vi "五参数水样测试.vi"(11 "启动参数":T1={"测量模式"="", "数据类型"="N"}) -> ()   [LabVIEW 2016, in "斯坦道原位多参数.lvlib"]
panel:
  in  "水温数据时间":timestamp
  out "Elapsed Time (s)":dbl caption="已用时间(s)"
  out "状态":string
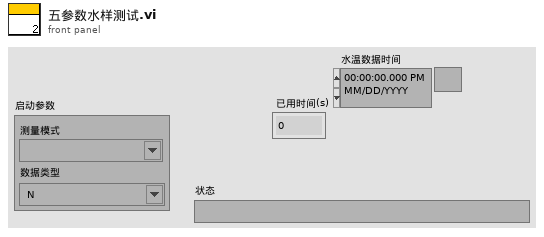
[diagram p1: front panel]
types:
  T1 = typedef "斯坦道原位多参数.lvlib/水样测试启动自定义输入参数.ctl" = cluster{"测量模式":string, "数据类型":string}
  T2 = cluster{"时间标识":timestamp, "设备":string, "日志信息":string, "流程参数":string}
  T3 = cluster{"水温":bool, "pH":bool, "DO":bool, "DOper":bool, "电导率":bool, "ORP":bool, "浊度":bool, "叶绿素a":bool, "藻密度":bool, "蓝绿藻":bool}
  T4 = typedef "原位多参数全参数字段定义.ctl" = cluster{"时间":timestamp, "水温":dbl, "pH":dbl, "DO":dbl, "DO%":dbl, "电导率":dbl, "ORP":dbl, "浊度":dbl, "叶绿素a":dbl, "藻密度":dbl, "蓝绿藻":dbl}
  T5 = cluster{"因子编码":string, "单位":string, "标样参考值":sgl, "水样数据时间":timestamp, "水样实测值":sgl, "水样数据标识":string, "K":sgl, "B":sgl, "T":sgl, "H":sgl, "水深":sgl, "探头温度":sgl, "信号值":sgl}
  T6 = cluster{"水温":dbl, "pH":dbl, "DO":dbl, "Cond":dbl, "Turb":dbl, "叶绿素":dbl, "藻密度":dbl, "蓝绿藻":dbl, "ORP":dbl, "NH3N":dbl}
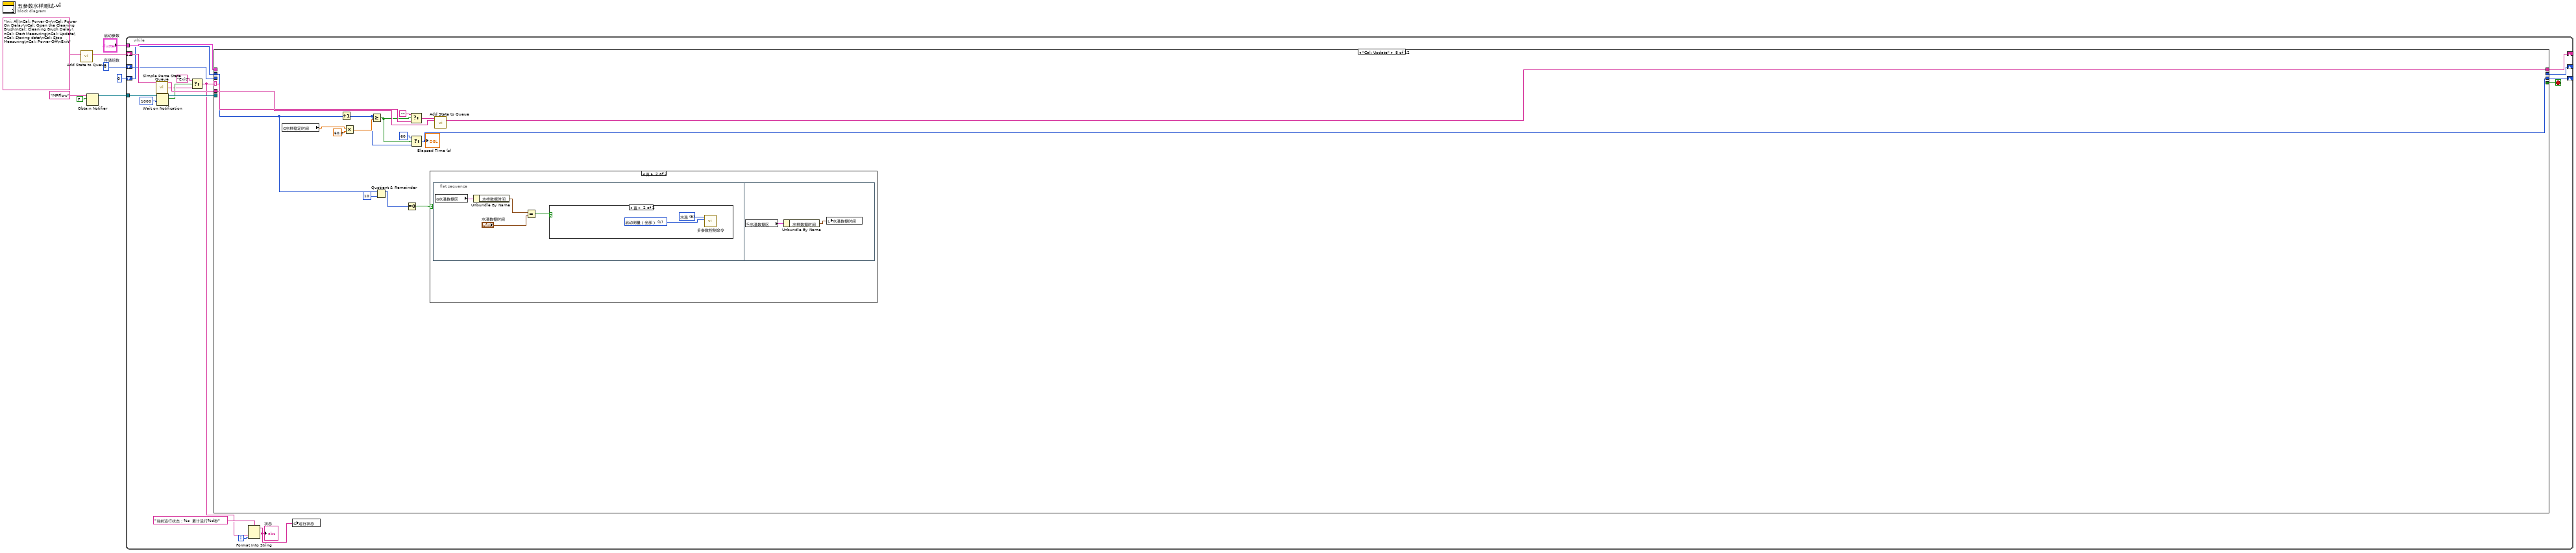
[diagram p0: block diagram]
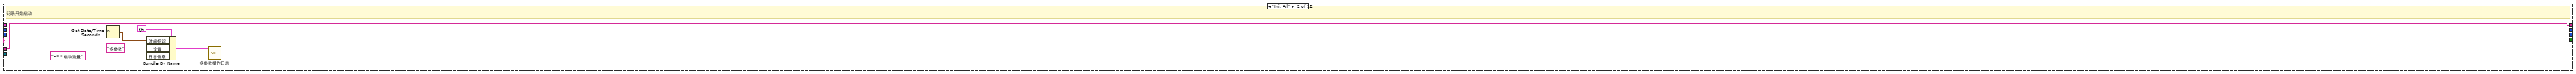
[diagram p3: hidden frame]
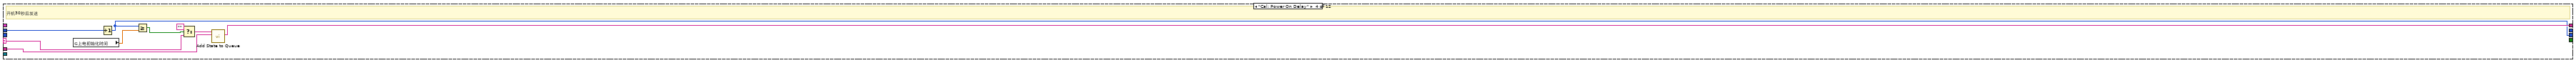
[diagram p5: hidden frame]
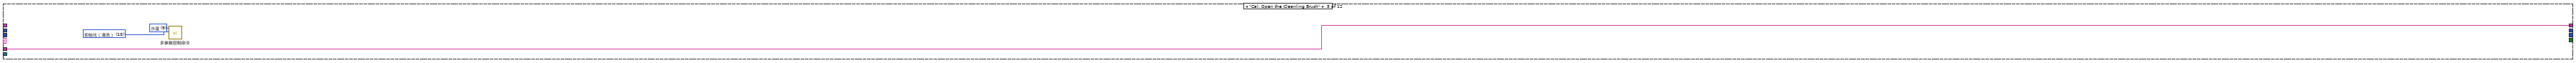
[diagram p6: hidden frame]
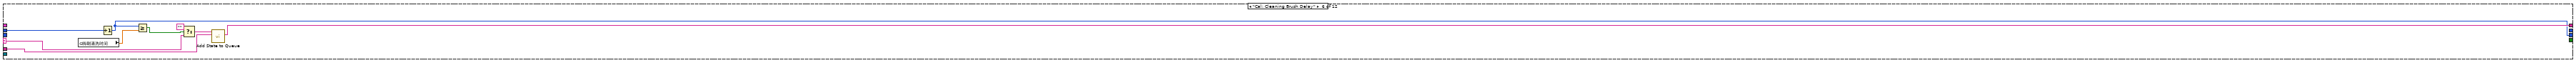
[diagram p7: hidden frame]
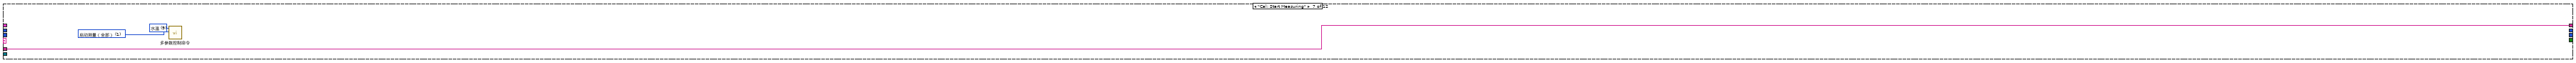
[diagram p8: hidden frame]
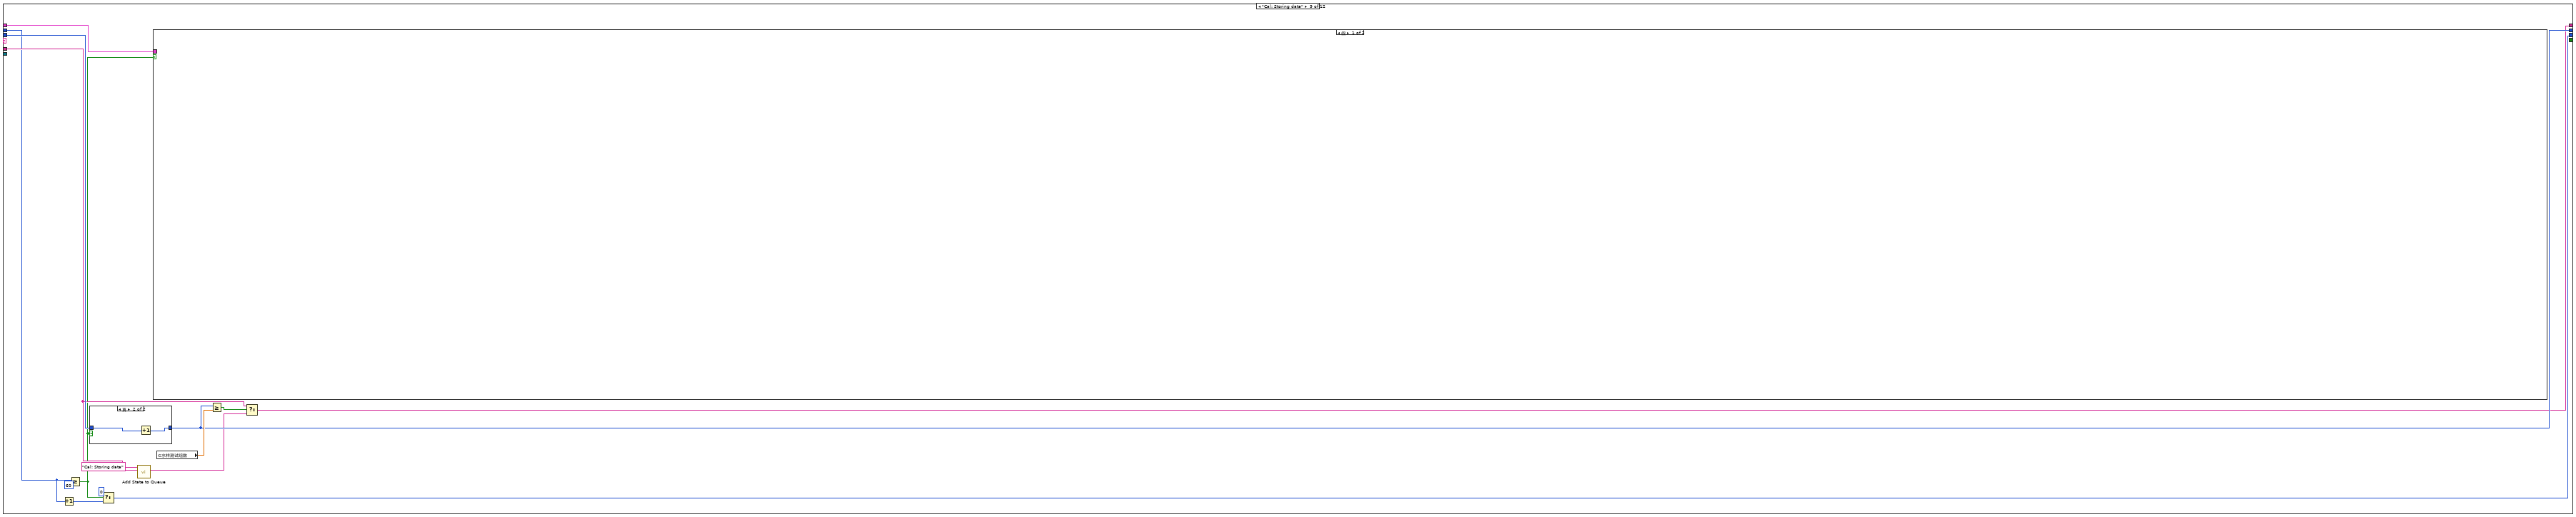
[diagram p11: hidden frame]
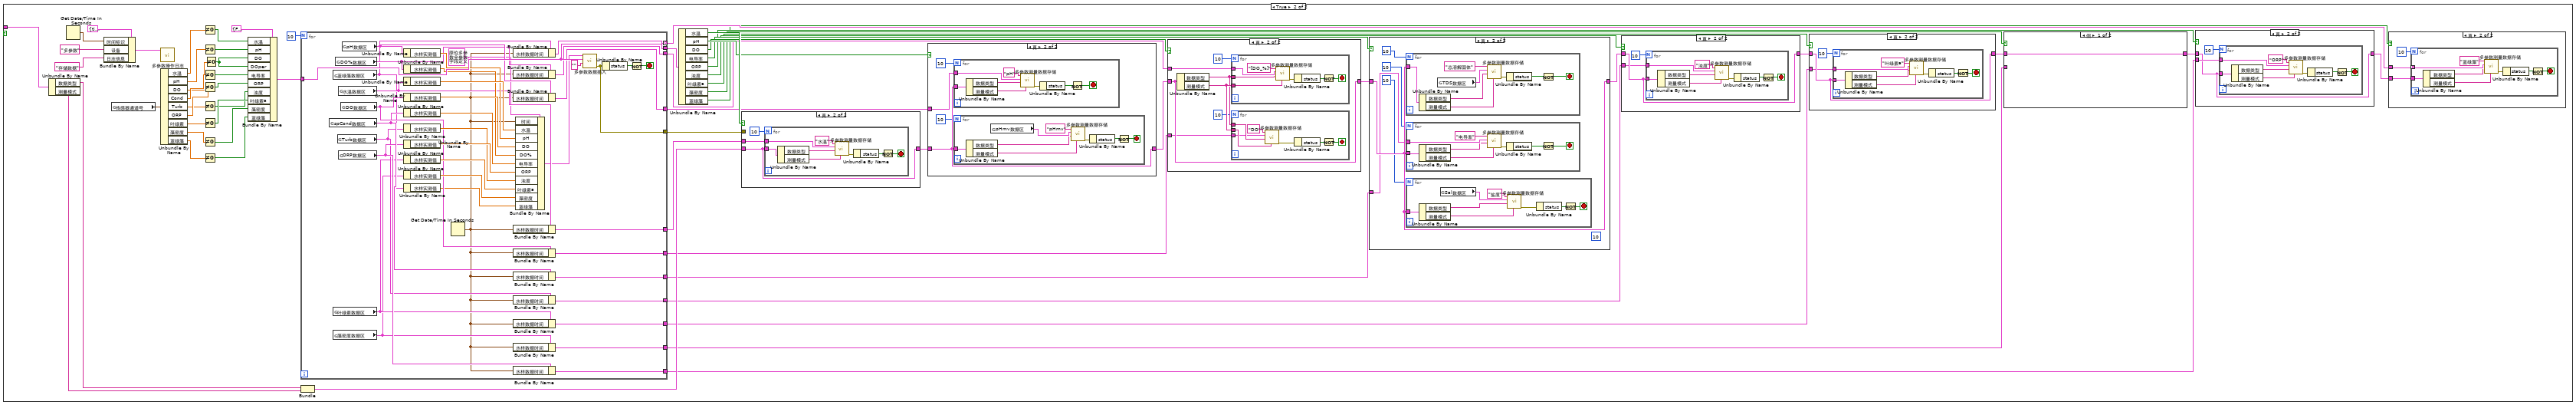
[diagram p13: hidden frame]
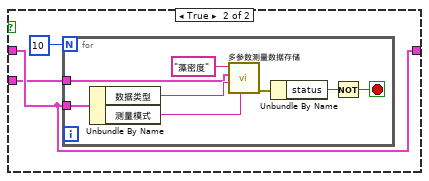
[diagram p16: hidden frame]
diagram:
  w1 = 0  # 存储组数
  n1 = call "Add State to Queue.vi"("State(s) In (\"\")"="Ini: All\nCal: Power On\nCal: Power On Delay\nCal: Open the Cleaning Brush\nCal: Cleaning Brush Delay\nCal: Start Measuring\nCal: Update\nCal: Storing data\nCal: Stop Measuring\nCal: Power Off\nExit" ("State(s) In (\"\")")) -> ("States Out"=w7:string)  [unwired: 14 in]
  n2 = Obtain Notifier(name (unnamed)="MPFlow" ("名称（未命名）"), notification data type=FALSE) -> (notifier out=w4:refnum<notifier>)  [unwired: 2 in, 2 out]
  n3 = while {
    shift-right: [w25] -> _
    shift-left: w7 -> [w27]
    tunnel: w4 -> [w24]
    tunnel: "启动参数" -> [w23]
    shift-right: [w11] -> _
    shift-left: 0 -> [w12]
    shift-right: [w10] -> _
    shift-left: w1 -> [w9]
    i -> [w21]
    stop <- w19 stop-if-true
    n4 = call "Simple Parse State Queue.vi"("State Queue"=w27) -> ("Remain States"=w26:string, "Next State"=w14:string)  [unwired: 13 in]
    n5 = Wait on Notification(notifier=w24, timeout in ms (-1)=1000 ("超时毫秒(-1)")) -> (notifier out=w18:refnum<notifier>, notification=w16:bool)  [unwired: 2 in, 2 out]
    n6 = Select(t="Exit" ("State(s) In (\"\")"), s=w16, f=w14) -> (s? t:f=w13:string)
    n7 = case shown="\"Cal: Update\"" w13 {
      selector: w13 -> [_ _ _ w42 _ w52 _ w73 _ _ _ _]
      tunnel: w26 -> [w28 w34 w35 w44 w47 w56 w57 w74 w90 w344 w353 w355]
      tunnel: [w28 w34 w35 w43 w47 w55 w57 w70 w92 w344 w353 w355] -> w25
      tunnel: w18 -> [_ _ _ _ _ _ _ _ _ _ _ w354]
      tunnel: w23 -> [_ _ _ _ _ _ _ _ w98 _ _ _]
      tunnel: [_ _ _ _ _ _ _ _ _ _ _ TRUE] -> w19
      tunnel: w12 -> [_ _ _ w39 _ w51 _ w63 w89 _ _ _]
      tunnel: [_ _ _ w38 _ w50 _ w65 w86 _ _ _] -> w11
      tunnel: w9 -> [_ _ _ _ _ _ _ _ w97 _ _ _]
      tunnel: [_ _ _ _ _ _ _ _ w94 _ _ _] -> w10
      frame Default {
      }
      frame "Ini: All" {
        # "记录开始启动"
        n8 = Get Date/Time In Seconds() -> (seconds since 1Jan1904=w30:timestamp)
        n9 = Bundle By Name(cluster=T2 {"时间标识"=timestamp(0 s since 1904-01-01), "设备"="", "日志信息"="", "流程参数"=""} ("data in"), "时间标识"=w30, "设备"="多参数", "日志信息"="-->>启动测量") -> (w31:T2)
        n10 = call "多参数操作日志.vi"("data"=w31) -> ()  [unwired: 10 in, 1 out]
      }
      frame "Cal: Power On" {
      }
      frame "Cal: Power On Delay" {
        # "开机30秒后发送"
        n11 = global read "多参数断电保存全局变量.vi" "上电初始化时间"() -> (w36:dbl)
        n12 = Increment(x=w39) -> (x+1=w38:i32)
        n13 = Greater Or Equal?(x=w38, y=w36) -> (x >= y?=w37:bool)
        n14 = Select(t="", s=w37, f=w42) -> (s? t:f=w40:string)
        n15 = call "Add State to Queue.vi"("State(s) In Front (\"\")"=w40, "State(s) In (\"\")"=w44) -> ("States Out"=w43:string)  [unwired: 13 in]
      }
      frame "Cal: Open the Cleanling Brush" {
        w46 = u16 10 items=["启动测量（全部）"=1, "初始化（清洗）"=10, "停止测量（全部）"=11, "校时"=13, "启动测量（单个传感器）"=19, "停止测量（单个传感器）"=20] ("控制命令")
        w45 = u16 9 items=["氨氮"=3, "水温"=9, "pH值"=10, "溶解氧"=11, "电导率"=12, "浊度"=13, "叶绿素a"=14, "藻密度"=15, "蓝绿藻"=16, "氧化还原电位"=17, "溶解氧%"=18, "盐度"=19] ("站号")
        n16 = call "多参数控制命令.vi"("控制命令"=w46, "站号"=w45) -> ()  [unwired: 9 in, 1 out]
      }
      frame "Cal: Cleaning Brush Delay" {
        n17 = global read "多参数断电保存全局变量.vi" "转刷清洗时间"() -> (w48:dbl)
        n18 = Increment(x=w51) -> (x+1=w50:i32)
        n19 = Greater Or Equal?(x=w50, y=w48) -> (x >= y?=w49:bool)
        n20 = Select(t="", s=w49, f=w52) -> (s? t:f=w53:string)
        n21 = call "Add State to Queue.vi"("State(s) In Front (\"\")"=w53, "State(s) In (\"\")"=w56) -> ("States Out"=w55:string)  [unwired: 13 in]
      }
      frame "Cal: Start Measuring" {
        w59 = u16 1 items=["启动测量（全部）"=1, "初始化（清洗）"=10, "停止测量（全部）"=11, "校时"=13, "启动测量（单个传感器）"=19, "停止测量（单个传感器）"=20] ("控制命令")
        w58 = u16 9 items=["氨氮"=3, "水温"=9, "pH值"=10, "溶解氧"=11, "电导率"=12, "浊度"=13, "叶绿素a"=14, "藻密度"=15, "蓝绿藻"=16, "氧化还原电位"=17, "溶解氧%"=18, "盐度"=19] ("站号")
        n22 = call "多参数控制命令.vi"("控制命令"=w59, "站号"=w58) -> ()  [unwired: 9 in, 1 out]
      }
      frame "Cal: Update" {
        n23 = global read "多参数断电保存全局变量.vi" "水样稳定时间"() -> (w68:dbl)
        n24 = Increment(x=w63) -> (x+1=w66:i32)
        n25 = Multiply(x=w68, y=60.0) -> (x*y=w69:dbl)
        n26 = Greater Or Equal?(x=w66, y=w69) -> (x >= y?=w67:bool)
        n27 = Quotient & Remainder(x=w63, y=10) -> (x-y*floor(x/y)=w61:i32)  [unwired: 1 out]
        n28 = Equal To 0?(x=w61) -> (x = 0?=w60:bool)
        n29 = Select(t="", s=w67, f=w73) -> (s? t:f=w72:string)
        n30 = Select(t=60, s=w67, f=w66) -> (s? t:f=w65:i32)
        "Elapsed Time (s)" <- w65
        n31 = case shown="真" w60 {
          frame False {
          }
          frame True {
            n32 = flat-sequence {
              frame #0 {
                n33 = global read "多参数全局变量.vi" "水温数据区"() -> (w79:T5)
                n34 = Unbundle By Name(w79) -> ("水样数据时间"=w78:timestamp)
                n35 = Equal?(x=w78, y="水温数据时间") -> (x = y?=w76:bool)
                n36 = case shown="真" w76 {
                  frame False {
                  }
                  frame True {
                    w80 = u16 1 items=["启动测量（全部）"=1, "初始化（清洗）"=10, "停止测量（全部）"=11, "校时"=13, "启动测量（单个传感器）"=19, "停止测量（单个传感器）"=20] ("控制命令")
                    w81 = u16 9 items=["氨氮"=3, "水温"=9, "pH值"=10, "溶解氧"=11, "电导率"=12, "浊度"=13, "叶绿素a"=14, "藻密度"=15, "蓝绿藻"=16, "氧化还原电位"=17, "溶解氧%"=18, "盐度"=19] ("站号")
                    n37 = call "多参数控制命令.vi"("控制命令"=w80, "站号"=w81) -> ()  [unwired: 9 in, 1 out]
                  }
                }
              }
              frame #1 {
                n38 = global read "多参数全局变量.vi" "水温数据区"() -> (w83:T5)
                n39 = Unbundle By Name(w83) -> ("水样数据时间"=w82:timestamp)
                n40 = local write "水温数据时间"(w82) -> ()
              }
            }
          }
        }
        n41 = call "Add State to Queue.vi"("State(s) In Front (\"\")"=w72, "State(s) In (\"\")"=w74) -> ("States Out"=w70:string)  [unwired: 13 in]
      }
      frame "Cal: Storing data" {
        n42 = Increment(x=w89) -> (x+1=w87:i32)
        n43 = Greater Or Equal?(x=w89, y=60) -> (x >= y?=w84:bool)
        n44 = case shown="真" w84 {
          tunnel: w97 -> [w99 w101]
          tunnel: [w99 w100] -> w94
          frame False {
          }
          frame True {
            n45 = Increment(x=w101) -> (x+1=w100:i32)
          }
        }
        n46 = Select(t=0, s=w84, f=w87) -> (s? t:f=w86:i32)
        n47 = call "Add State to Queue.vi"("State(s) In Front (\"\")"="Cal: Storing data" ("State(s) In Front (\"\")"), "State(s) In (\"\")"=w90) -> ("States Out"=w91:string)  [unwired: 13 in]
        n48 = case shown="假" w84 {
          tunnel: w98 -> [_ w147]
          frame False {
          }
          frame True {
            n49 = Unbundle By Name(w147) -> ("数据类型"=w148:string, "测量模式"=w149:string)
            n50 = Get Date/Time In Seconds() -> (seconds since 1Jan1904=w156:timestamp)
            n51 = Bundle By Name(cluster=T2 {"时间标识"=timestamp(0 s since 1904-01-01), "设备"="", "日志信息"="", "流程参数"=""} ("data in"), "时间标识"=w156, "设备"="多参数", "日志信息"="存储数据") -> (w157:T2)
            n52 = global read "多参数全局变量.vi" "传感器通道号"() -> (w129:T6)
            n53 = call "多参数操作日志.vi"("data"=w157) -> ()  [unwired: 10 in, 1 out]
            n54 = Unbundle By Name(w129) -> ("水温"=w127:dbl, "pH"=w130:dbl, "DO"=w132:dbl, "Cond"=w134:dbl, "Turb"=w136:dbl, "ORP"=w138:dbl, "叶绿素"=w140:dbl, "藻密度"=w141:dbl, "蓝绿藻"=w106:dbl)
            n55 = Not Equal To 0?(x=w127) -> (x != 0?=w128:bool)
            n56 = Not Equal To 0?(x=w130) -> (x != 0?=w131:bool)
            n57 = Not Equal To 0?(x=w134) -> (x != 0?=w135:bool)
            n58 = Not Equal To 0?(x=w138) -> (x != 0?=w139:bool)
            n59 = Not Equal To 0?(x=w136) -> (x != 0?=w137:bool)
            n60 = Not Equal To 0?(x=w140) -> (x != 0?=w142:bool)
            n61 = Not Equal To 0?(x=w141) -> (x != 0?=w143:bool)
            n62 = Not Equal To 0?(x=w106) -> (x != 0?=w105:bool)
            n63 = Not Equal To 0?(x=w132) -> (x != 0?=w133:bool)
            n64 = Bundle By Name(cluster=T3 {"水温"=FALSE, "pH"=FALSE, "DO"=FALSE, "DOper"=FALSE, "电导率"=FALSE, "ORP"=FALSE, "浊度"=FALSE, "叶绿素a"=FALSE, "藻密度"=FALSE, "蓝绿藻"=FALSE} ("columns enable"), "水温"=w128, "pH"=w131, "DO"=w133, "DOper"=w133, "电导率"=w135, "ORP"=w139, "浊度"=w137, "叶绿素a"=w142, "藻密度"=w143, "蓝绿藻"=w105) -> (w126:T3)
            n65 = for {
              N: 10 -> [_]
              tunnel: [w208] -> w144
              tunnel: w126 -> [w207]
              tunnel: [w207] -> w117
              tunnel: [w183] -> w116
              tunnel: [w182] -> w115
              tunnel: [w181] -> w114
              tunnel: [w184] -> w113
              tunnel: [w180] -> w112
              tunnel: [w188] -> w111
              tunnel: [w185] -> w110
              tunnel: [w186] -> w109
              tunnel: [w187] -> w108
              tunnel: [w173] -> w103 mode=indexing
              stop <- w209 stop-if-true
              n66 = global read "多参数全局变量.vi" "spCond数据区"() -> (w193:T5)
              n67 = global read "多参数全局变量.vi" "蓝绿藻数据区"() -> (w175:T5)
              n68 = global read "多参数全局变量.vi" "叶绿素数据区"() -> (w190:T5)
              n69 = global read "多参数全局变量.vi" "藻密度数据区"() -> (w189:T5)
              n70 = global read "多参数全局变量.vi" "DO%数据区"() -> (w194:T5)
              n71 = global read "多参数全局变量.vi" "Turb数据区"() -> (w191:T5)
              n72 = global read "多参数全局变量.vi" "水温数据区"() -> (w197:T5)
              n73 = global read "多参数全局变量.vi" "ORP数据区"() -> (w192:T5)
              n74 = global read "多参数全局变量.vi" "DO数据区"() -> (w195:T5)
              n75 = global read "多参数全局变量.vi" "pH数据区"() -> (w196:T5)
              n76 = Unbundle By Name(w196) -> ("水样实测值"=w205:sgl)
              n77 = Unbundle By Name(w194) -> ("水样实测值"=w203:sgl)
              n78 = Unbundle By Name(w197) -> ("水样实测值"=w206:sgl)
              n79 = Unbundle By Name(w195) -> ("水样实测值"=w204:sgl)
              n80 = Unbundle By Name(w193) -> ("水样实测值"=w202:sgl)
              n81 = Unbundle By Name(w191) -> ("水样实测值"=w200:sgl)
              n82 = Unbundle By Name(w192) -> ("水样实测值"=w201:sgl)
              n83 = Unbundle By Name(w190) -> ("水样实测值"=w199:sgl)
              n84 = Unbundle By Name(w189) -> ("水样实测值"=w198:sgl)
              n85 = Unbundle By Name(w175) -> ("水样实测值"=w176:sgl)
              n86 = Get Date/Time In Seconds() -> (seconds since 1Jan1904=w174:timestamp)
              n87 = Bundle By Name(cluster=w175, "水样数据时间"=w174) -> (w173:T5)
              n88 = Bundle By Name(cluster=w194, "水样数据时间"=w174) -> (w184:T5)
              n89 = Bundle By Name(cluster=w196, "水样数据时间"=w174) -> (w182:T5)
              n90 = Bundle By Name(cluster=w197, "水样数据时间"=w174) -> (w183:T5)
              n91 = Bundle By Name(cluster=w195, "水样数据时间"=w174) -> (w181:T5)
              n92 = Bundle By Name(cluster=w193, "水样数据时间"=w174) -> (w180:T5)
              n93 = Bundle By Name(cluster=w191, "水样数据时间"=w174) -> (w185:T5)
              n94 = Bundle By Name(cluster=w190, "水样数据时间"=w174) -> (w186:T5)
              n95 = Bundle By Name(cluster=w189, "水样数据时间"=w174) -> (w187:T5)
              n96 = Bundle By Name(cluster=w192, "水样数据时间"=w174) -> (w188:T5)
              n97 = Bundle By Name(cluster=T4 {"时间"=timestamp(0 s since 1904-01-01), "水温"=0.0, "pH"=0.0, "DO"=0.0, "DO%"=0.0, "电导率"=0.0, "ORP"=0.0, "浊度"=0.0, "叶绿素a"=0.0, "藻密度"=0.0, "蓝绿藻"=0.0} ("data in"), "时间"=w174, "水温"=w206, "pH"=w205, "DO"=w204, "DO%"=w203, "电导率"=w202, "ORP"=w201, "浊度"=w200, "叶绿素a"=w199, "藻密度"=w198, "蓝绿藻"=w176) -> (w178:T4)
              n98 = call "多参数数据插入.vi"("编号"="", "columns enable"=w207, "data in"=w178) -> ("error out"=w208:errorcluster)  [unwired: 8 in]
              n99 = Unbundle By Name(w208) -> ("status"=w210:bool)
              n100 = Not(x=w210) -> (.not. x?=w209:bool)
            }
            n101 = Bundle("数据类型"=w148, "测量模式"=w149) -> (w150:cluster{"数据类型":string, "测量模式":string})  [unwired: 1 in]
            n102 = Unbundle By Name(w117) -> ("水温"=w125:bool, "pH"=w124:bool, "DO"=w123:bool, "电导率"=w122:bool, "ORP"=w118:bool, "浊度"=w121:bool, "叶绿素a"=w120:bool, "藻密度"=w119:bool, "蓝绿藻"=w102:bool)
            n103 = case shown="真" w125 {
              tunnel: w150 -> [w332 w335]
              tunnel: [w332 w335] -> w151
              tunnel: w144 -> [_ _]
              tunnel: w116 -> [_ w333]
              frame False {
              }
              frame True {
                n104 = for {
                  N: 10 -> [_]
                  tunnel: w335 -> [w343]
                  tunnel: w333 -> [w338]
                  stop <- w340 stop-if-true
                  n105 = Unbundle By Name(w343) -> ("数据类型"=w337:string, "测量模式"=w336:string)
                  n106 = call "多参数测量数据存储.vi"("测量模式"=w336, "数据类型"=w337, "数据区"=w338, "table输入"="水温") -> ("error out"=w342:errorcluster)  [unwired: 7 in]
                  n107 = Unbundle By Name(w342) -> ("status"=w341:bool)
                  n108 = Not(x=w341) -> (.not. x?=w340:bool)
                }
              }
            }
            n109 = case shown="真" w124 {
              tunnel: w151 -> [w311 w315]
              tunnel: [w311 w315] -> w153
              tunnel: w115 -> [_ w312]
              frame False {
              }
              frame True {
                n110 = for {
                  N: 10 -> [_]
                  tunnel: w315 -> [w331]
                  tunnel: w312 -> [w324]
                  stop <- w328 stop-if-true
                  n111 = Unbundle By Name(w331) -> ("数据类型"=w326:string, "测量模式"=w325:string)
                  n112 = call "多参数测量数据存储.vi"("测量模式"=w325, "数据类型"=w326, "数据区"=w324, "table输入"="pH") -> ("error out"=w330:errorcluster)  [unwired: 7 in]
                  n113 = Unbundle By Name(w330) -> ("status"=w329:bool)
                  n114 = Not(x=w329) -> (.not. x?=w328:bool)
                }
                n115 = for {
                  N: 10 -> [_]
                  tunnel: w315 -> [w323]
                  stop <- w320 stop-if-true
                  n116 = Unbundle By Name(w323) -> ("数据类型"=w317:string, "测量模式"=w316:string)
                  n117 = global read "多参数全局变量.vi" "pHmv数据区"() -> (w318:T5)
                  n118 = call "多参数测量数据存储.vi"("测量模式"=w316, "数据类型"=w317, "数据区"=w318, "table输入"="pHmv") -> ("error out"=w322:errorcluster)  [unwired: 7 in]
                  n119 = Unbundle By Name(w322) -> ("status"=w321:bool)
                  n120 = Not(x=w321) -> (.not. x?=w320:bool)
                }
              }
            }
            n121 = case shown="真" w123 {
              tunnel: [w289 w296] -> w152
              tunnel: w153 -> [w289 w296]
              tunnel: w114 -> [_ w291]
              tunnel: w113 -> [_ w290]
              frame False {
              }
              frame True {
                n122 = Unbundle By Name(w296) -> ("数据类型"=w294:string, "测量模式"=w295:string)
                n123 = for {
                  N: 10 -> [_]
                  tunnel: w295 -> [w304]
                  tunnel: w294 -> [w305]
                  tunnel: w290 -> [w306]
                  stop <- w308 stop-if-true
                  n124 = call "多参数测量数据存储.vi"("测量模式"=w304, "数据类型"=w305, "数据区"=w306, "table输入"="[DO_%]") -> ("error out"=w310:errorcluster)  [unwired: 7 in]
                  n125 = Unbundle By Name(w310) -> ("status"=w309:bool)
                  n126 = Not(x=w309) -> (.not. x?=w308:bool)
                }
                n127 = for {
                  N: 10 -> [_]
                  tunnel: w295 -> [w298]
                  tunnel: w294 -> [w299]
                  tunnel: w291 -> [w297]
                  stop <- w301 stop-if-true
                  n128 = call "多参数测量数据存储.vi"("测量模式"=w298, "数据类型"=w299, "数据区"=w297, "table输入"="DO") -> ("error out"=w303:errorcluster)  [unwired: 7 in]
                  n129 = Unbundle By Name(w303) -> ("status"=w302:bool)
                  n130 = Not(x=w302) -> (.not. x?=w301:bool)
                }
              }
            }
            n131 = case shown="真" w122 {
              tunnel: w152 -> [w259 w264]
              tunnel: [w259 w264] -> w154
              tunnel: w112 -> [_ w260]
              frame False {
              }
              frame True {
                (unwired) 10
                n132 = for {
                  N: 10 -> [_]
                  tunnel: w264 -> [w272]
                  stop <- w269 stop-if-true
                  n133 = Unbundle By Name(w272) -> ("数据类型"=w266:string, "测量模式"=w265:string)
                  n134 = global read "多参数全局变量.vi" "TDS数据区"() -> (w267:T5)
                  n135 = call "多参数测量数据存储.vi"("测量模式"=w265, "数据类型"=w266, "数据区"=w267, "table输入"="总溶解固体") -> ("error out"=w271:errorcluster)  [unwired: 7 in]
                  n136 = Unbundle By Name(w271) -> ("status"=w270:bool)
                  n137 = Not(x=w270) -> (.not. x?=w269:bool)
                }
                n138 = for {
                  N: 10 -> [_]
                  tunnel: w264 -> [w280]
                  tunnel: w260 -> [w275]
                  stop <- w277 stop-if-true
                  n139 = Unbundle By Name(w280) -> ("数据类型"=w274:string, "测量模式"=w273:string)
                  n140 = call "多参数测量数据存储.vi"("测量模式"=w273, "数据类型"=w274, "数据区"=w275, "table输入"="电导率") -> ("error out"=w279:errorcluster)  [unwired: 7 in]
                  n141 = Unbundle By Name(w279) -> ("status"=w278:bool)
                  n142 = Not(x=w278) -> (.not. x?=w277:bool)
                }
                n143 = for {
                  N: 10 -> [_]
                  tunnel: w264 -> [w288]
                  stop <- w285 stop-if-true
                  n144 = Unbundle By Name(w288) -> ("数据类型"=w282:string, "测量模式"=w281:string)
                  n145 = global read "多参数全局变量.vi" "Sal数据区"() -> (w283:T5)
                  n146 = call "多参数测量数据存储.vi"("测量模式"=w281, "数据类型"=w282, "数据区"=w283, "table输入"="盐度") -> ("error out"=w287:errorcluster)  [unwired: 7 in]
                  n147 = Unbundle By Name(w287) -> ("status"=w286:bool)
                  n148 = Not(x=w286) -> (.not. x?=w285:bool)
                }
              }
            }
            n149 = case shown="真" w121 {
              tunnel: w154 -> [w247 w250]
              tunnel: [w247 w250] -> w160
              tunnel: w110 -> [_ w248]
              frame False {
              }
              frame True {
                n150 = for {
                  N: 10 -> [_]
                  tunnel: w250 -> [w258]
                  tunnel: w248 -> [w253]
                  stop <- w255 stop-if-true
                  n151 = Unbundle By Name(w258) -> ("数据类型"=w252:string, "测量模式"=w251:string)
                  n152 = call "多参数测量数据存储.vi"("测量模式"=w251, "数据类型"=w252, "数据区"=w253, "table输入"="浊度") -> ("error out"=w257:errorcluster)  [unwired: 7 in]
                  n153 = Unbundle By Name(w257) -> ("status"=w256:bool)
                  n154 = Not(x=w256) -> (.not. x?=w255:bool)
                }
              }
            }
            n155 = case shown="真" w120 {
              tunnel: w160 -> [w235 w238]
              tunnel: [w235 w238] -> w161
              tunnel: w109 -> [_ w236]
              frame False {
              }
              frame True {
                n156 = for {
                  N: 10 -> [_]
                  tunnel: w238 -> [w246]
                  tunnel: w236 -> [w239]
                  stop <- w243 stop-if-true
                  n157 = Unbundle By Name(w246) -> ("数据类型"=w242:string, "测量模式"=w241:string)
                  n158 = call "多参数测量数据存储.vi"("测量模式"=w241, "数据类型"=w242, "数据区"=w239, "table输入"="叶绿素a") -> ("error out"=w245:errorcluster)  [unwired: 7 in]
                  n159 = Unbundle By Name(w245) -> ("status"=w244:bool)
                  n160 = Not(x=w244) -> (.not. x?=w243:bool)
                }
              }
            }
            n161 = case shown="假" w119 {
              tunnel: w161 -> [w223 w226]
              tunnel: [w223 w226] -> w146
              tunnel: w108 -> [_ w224]
              frame False {
              }
              frame True {
                n162 = for {
                  N: 10 -> [_]
                  tunnel: w226 -> [w234]
                  tunnel: w224 -> [w227]
                  stop <- w231 stop-if-true
                  n163 = Unbundle By Name(w234) -> ("数据类型"=w229:string, "测量模式"=w228:string)
                  n164 = call "多参数测量数据存储.vi"("测量模式"=w228, "数据类型"=w229, "数据区"=w227, "table输入"="藻密度") -> ("error out"=w233:errorcluster)  [unwired: 7 in]
                  n165 = Unbundle By Name(w233) -> ("status"=w232:bool)
                  n166 = Not(x=w232) -> (.not. x?=w231:bool)
                }
              }
            }
            n167 = case shown="真" w118 {
              tunnel: w146 -> [w211 w212]
              tunnel: w111 -> [_ w213]
              tunnel: [w211 w212] -> w104
              frame False {
              }
              frame True {
                n168 = for {
                  N: 10 -> [_]
                  tunnel: w212 -> [w222]
                  tunnel: w213 -> [w217]
                  stop <- w219 stop-if-true
                  n169 = Unbundle By Name(w222) -> ("数据类型"=w216:string, "测量模式"=w215:string)
                  n170 = call "多参数测量数据存储.vi"("测量模式"=w215, "数据类型"=w216, "数据区"=w217, "table输入"="ORP") -> ("error out"=w221:errorcluster)  [unwired: 7 in]
                  n171 = Unbundle By Name(w221) -> ("status"=w220:bool)
                  n172 = Not(x=w220) -> (.not. x?=w219:bool)
                }
              }
            }
            n173 = case shown="真" w102 {
              tunnel: w104 -> [_ w164]
              tunnel: w103 -> [_ w162]
              frame False {
              }
              frame True {
                n174 = for {
                  N: 10 -> [_]
                  tunnel: w164 -> [w172]
                  tunnel: w162 -> [w167] mode=indexing
                  stop <- w169 stop-if-true
                  n175 = Unbundle By Name(w172) -> ("数据类型"=w166:string, "测量模式"=w165:string)
                  n176 = call "多参数测量数据存储.vi"("测量模式"=w165, "数据类型"=w166, "数据区"=w167, "table输入"="蓝绿藻") -> ("error out"=w171:errorcluster)  [unwired: 7 in]
                  n177 = Unbundle By Name(w171) -> ("status"=w170:bool)
                  n178 = Not(x=w170) -> (.not. x?=w169:bool)
                }
              }
            }
          }
        }
        n179 = global read "多参数断电保存全局变量.vi" "水样测试组数"() -> (w95:dbl)
        n180 = Greater Or Equal?(x=w94, y=w95) -> (x >= y?=w93:bool)
        n181 = Select(t=w90, s=w93, f=w91) -> (s? t:f=w92:string)
      }
      frame "Cal: Stop Measuring" {
        n182 = flat-sequence {
          frame #0 {
            w350 = u16 11 items=["启动测量（全部）"=1, "初始化（清洗）"=10, "停止测量（全部）"=11, "校时"=13, "启动测量（单个传感器）"=19, "停止测量（单个传感器）"=20] ("控制命令")
            w351 = u16 9 items=["氨氮"=3, "水温"=9, "pH值"=10, "溶解氧"=11, "电导率"=12, "浊度"=13, "叶绿素a"=14, "藻密度"=15, "蓝绿藻"=16, "氧化还原电位"=17, "溶解氧%"=18, "盐度"=19] ("站号")
            n183 = call "多参数控制命令.vi"("控制命令"=w350, "站号"=w351) -> ()  [unwired: 9 in, 1 out]
          }
          frame #1 {
            n184 = Wait (ms)(milliseconds to wait=u32 2000 ("等待时间（毫秒）")) -> ()  [unwired: 1 out]
          }
        }
        n185 = Get Date/Time In Seconds() -> (seconds since 1Jan1904=w347:timestamp)
        n186 = Bundle By Name(cluster=T2 {"时间标识"=timestamp(0 s since 1904-01-01), "设备"="", "日志信息"="", "流程参数"=""} ("data in"), "时间标识"=w347, "设备"="多参数", "日志信息"="-->>停止测量") -> (w346:T2)
        n187 = call "多参数操作日志.vi"("data"=w346) -> ()  [unwired: 10 in, 1 out]
      }
      frame "Cal: Power Off" {
      }
      frame "Exit" {
        n188 = Release Notifier(notifier=w354) -> ()  [unwired: 2 in, 3 out]
      }
    }
    n189 = Format Into String(format string="当前运行状态：%s  累计运行%d秒" ("格式字符串"), w13, w21) -> (resulting string=w20:string)  [unwired: 2 in, 1 out]
    "状态" <- w20
    n190 = global write "多参数全局变量.vi" "运行状态"(w20) -> ()
  }
